vi "SubDaqInit.vi"(8 "error in (no error)":errorcluster, 9 "SubQueueIN":refnum<queue>, 10 "MainQueueIN":refnum<queue>, 11 "Data Value Reference IN":refnum<data-value>) -> (0 "error out":errorcluster, 3 "Data Value Reference out":refnum<data-value>)   [LabVIEW 2013]
uses:
  Control/SystemCommand.ctl
  Control/SystemData.ctl
  Control/SignalType.ctl
  Control/SubDaqCommand.ctl
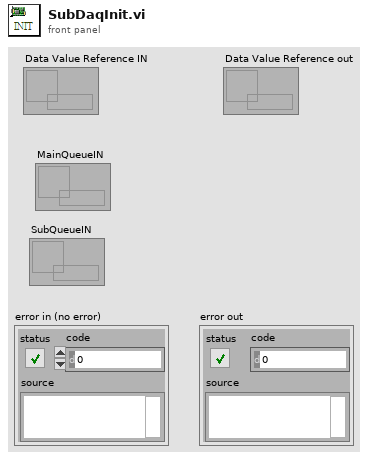
[diagram p1: front panel]
types:
  T1 = typedef "SystemCommand.ctl" = enum16{"None", "Init", "Close", "ShowNumeric", "ShowString", "ShowBool", "SquareNumeric", "ReverseString", "InvertBool", "FFT"}
  T2 = typedef "SubDaqCommand.ctl" = enum16{"None", "Init", "Work", "Stop", "Close"}
  T3 = typedef "SystemData.ctl" = cluster{"Numeric":dbl, "String":string, "Boolean":bool, "Frequency":dbl, "Amplitude":dbl, "SignalType":T4, "WaveformArray":waveform(dbl)[], "Reset":bool, "StateString":string, "FFTmagnitudes":cluster{"f0":dbl, "df":dbl, "magnitude":dbl[]}[]}
  T4 = typedef "SignalType.ctl" = enum16{"Sin", "Triangle", "Square"}
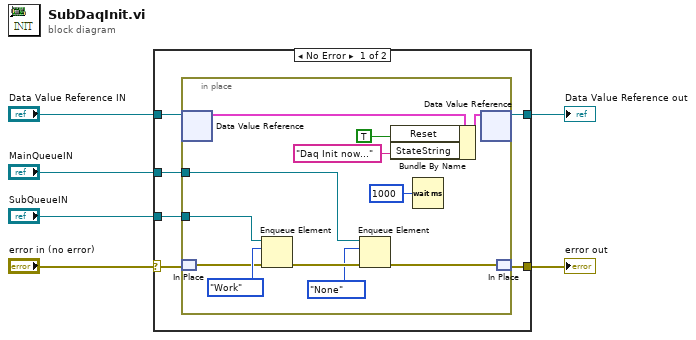
[diagram p0: block diagram]
diagram:
  n1 = case shown="No Error" "error in (no error)" {
    selector: "error in (no error)" -> [w10 w25]
    tunnel: "Data Value Reference IN" -> [w12 w26]
    tunnel: [w11 w26] -> w3
    tunnel: [w9 w25] -> w5
    tunnel: "MainQueueIN" -> [w8 _]
    tunnel: "SubQueueIN" -> [w7 _]
    frame No Error {
      n2 = in-place {
        in-place-border: w8 -> [w18]
        in-place-border: w7 -> [w23]
        n3 = in-place-dvr #1(w12) -> (w22:T3)  [unwired: 1 out]
        n4 = in-place-match #2(w10) -> (w19:errorcluster)
        n5 = Enqueue Element(queue=w23, element=SubDaqCommand."Work", error in (no error)=w19) -> (error out=w17:errorcluster)  [unwired: 1 in, 2 out]
        n6 = Enqueue Element(queue=w18, element=SystemCommand."None", error in (no error)=w17) -> (error out=w16:errorcluster)  [unwired: 1 in, 2 out]
        n7 = Bundle By Name(cluster=w22, "Reset"=TRUE, "StateString"="Daq Init now...") -> (w21:T3)
        n8 = Wait (ms)(milliseconds to wait=u32 1000) -> ()  [unwired: 1 out]
        n9 = in-place-dvr #1(w21) -> (w11:refnum<data-value>)  [unwired: 1 out]
        n10 = in-place-match #2(w16) -> (w9:errorcluster)
      }
    }
    frame Error {
    }
  }
  "error out" <- w5
  "Data Value Reference out" <- w3
